vi "combineZip.vi"(0 "basicPath":path, 5 "zipArray":path[](array[path]), 7 "combinedZip":path, 9 "status":refnum<vi>, 11 "错误输入":errorcluster) -> (4 "combinedZip out":path, 15 "error IO":errorcluster)   [LabVIEW 2011]
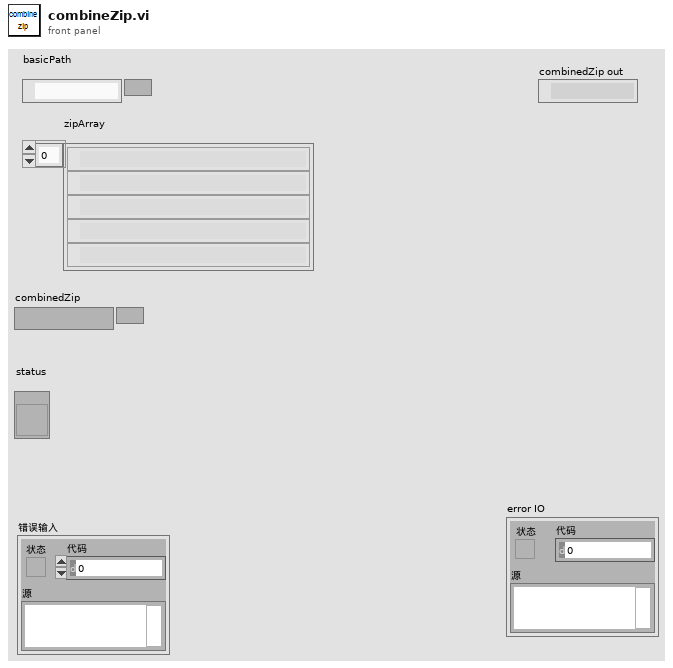
[diagram p1: front panel]
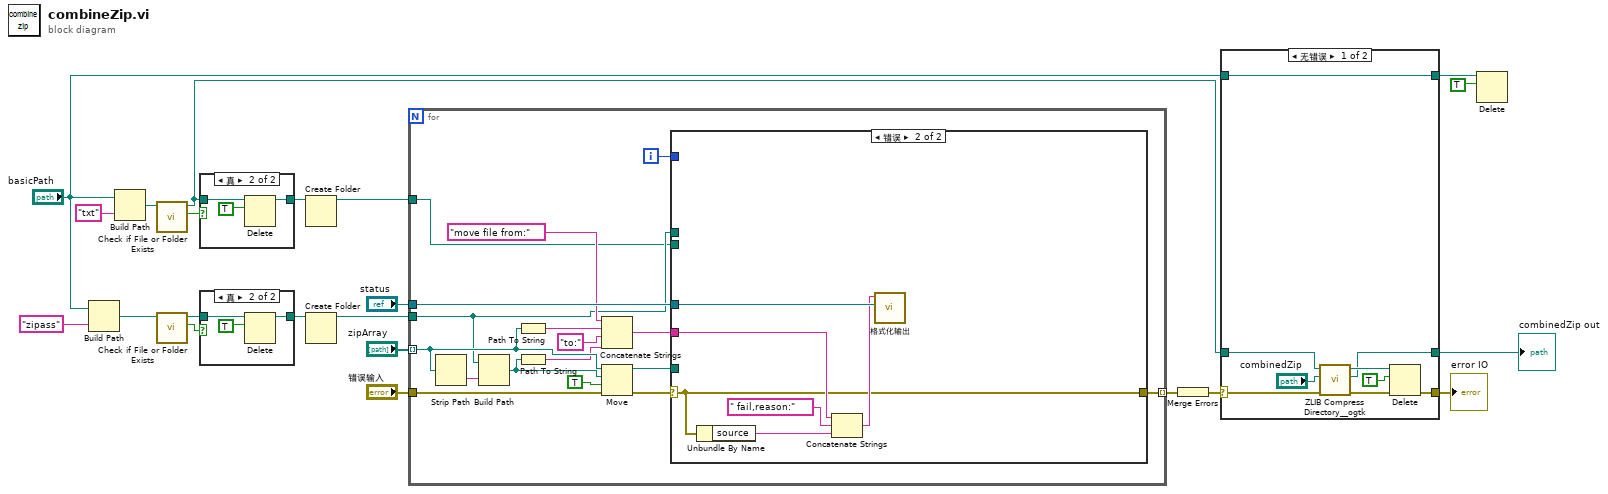
[diagram p0: block diagram]
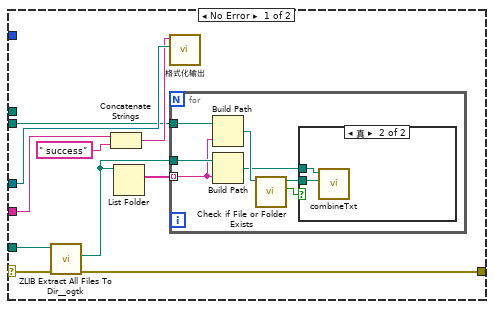
[diagram p5: hidden frame]
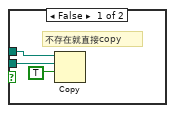
[diagram p6: hidden frame]
diagram:
  n1 = Build Path(base path="basicPath", name or relative path="zipass" ("名称或相对路径")) -> (appended path=w16:path)
  n2 = Build Path(base path="basicPath", name or relative path="txt" ("名称或相对路径")) -> (appended path=w11:path)
  n3 = call <vilib>:"Check if File or Folder Exists.vi"("path"=w11) -> ("file or folder exists?"=w13:bool, "dup path"=w7:path)  [unwired: 8 in, 1 out]
  n4 = call <vilib>:"Check if File or Folder Exists.vi"("path"=w16) -> ("file or folder exists?"=w20:bool, "dup path"=w19:path)  [unwired: 8 in, 1 out]
  n5 = case shown="真" w13 {
    tunnel: w7 -> [w23 w26]
    tunnel: [w23 w24] -> w12
    frame False {
    }
    frame True {
      n6 = Delete(path (use dialog)=w26, entire hierarchy (F)=TRUE ("整个层次结构(F)")) -> (deleted path=w24:path)  [unwired: 3 in, 2 out]
    }
  }
  n7 = case shown="真" w20 {
    tunnel: w19 -> [w27 w30]
    tunnel: [w27 w28] -> w18
    frame False {
    }
    frame True {
      n8 = Delete(path (use dialog)=w30, entire hierarchy (F)=TRUE ("整个层次结构(F)")) -> (deleted path=w28:path)  [unwired: 3 in, 2 out]
    }
  }
  n9 = Create Folder(path (use dialog)=w12) -> (created path=w10:path)  [unwired: 2 in, 2 out]
  n10 = Create Folder(path (use dialog)=w18) -> (created path=w17:path)  [unwired: 2 in, 2 out]
  n11 = for {
    tunnel: "zipArray" -> [w42] mode=indexing
    tunnel: w17 -> [w34]
    tunnel: "status" -> [w43]
    tunnel: "错误输入" -> [w35]
    tunnel: [w32] -> w9 mode=indexing
    tunnel: w10 -> [w31]
    i -> [w33]
    n12 = Strip Path(path=w42) -> (name=w47:string)  [unwired: 1 out]
    n13 = Build Path(base path=w34, name or relative path=w47) -> (appended path=w41:path)
    n14 = Path To String(path=w42) -> (string=w39:string)
    n15 = Path To String(path=w41) -> (string=w37:string)
    n16 = Concatenate Strings("move file from:" ("字符串"), w39, "to:" ("字符串"), w37) -> (w36:string)
    n17 = Move(source path=w42, error in=w35, 9:TRUE ("覆盖(F)"), 10:w41) -> (error out=w45:errorcluster, 3:w44:path)  [unwired: 1 in, 1 out]
    n18 = case shown="错误" w45 {
      selector: w45 -> [w52 w70]
      tunnel: w44 -> [w57 _]
      tunnel: w43 -> [w56 w72]
      tunnel: w36 -> [w55 w75]
      tunnel: w34 -> [_ _]
      tunnel: w33 -> [_ _]
      tunnel: [w51 w70] -> w32
      tunnel: w31 -> [w48 _]
      frame No Error {
        n19 = call <userlib>:"ZLIB Extract All Files To Dir__ogtk.vi"("error in (no error)"=w52, "archive name (file dialog)"=w57) -> ("error out"=w51:errorcluster, "root directory out"=w49:path)  [unwired: 7 in, 1 out]
        n20 = Concatenate Strings(w55, " success" ("字符串")) -> (w53:string)
        n21 = List Folder(path=w49) -> (filenames=w50:string[])  [unwired: 3 in, 3 out]
        n22 = call "格式化输出.vi"("字符串引用"=w56, "字符串"=w53) -> ()  [unwired: 9 in, 1 out]
        n23 = for {
          tunnel: w50 -> [w62] mode=indexing
          tunnel: w49 -> [w64]
          tunnel: w48 -> [w63]
          n24 = Build Path(base path=w63, name or relative path=w62) -> (appended path=w61:path)
          n25 = Build Path(base path=w64, name or relative path=w62) -> (appended path=w59:path)
          n26 = call <vilib>:"Check if File or Folder Exists.vi"("path"=w61) -> ("file or folder exists?"=w60:bool, "dup path"=w58:path)  [unwired: 8 in, 1 out]
          n27 = case shown="真" w60 {
            tunnel: w59 -> [w67 w69]
            tunnel: w58 -> [w66 w68]
            frame False {
              # "不存在就直接copy"
              n28 = Copy(9:TRUE ("覆盖(F)"), 10:w66, 11:w67) -> ()  [unwired: 2 in, 3 out]
            }
            frame True {
              n29 = call "combineTxt.vi"("parentPath"=w68, "childPath"=w69) -> ()  [unwired: 9 in, 1 out]
            }
          }
        }
      }
      frame Error {
        n30 = Unbundle By Name(w70) -> ("source"=w73:string)
        n31 = Concatenate Strings(w75, " fail,reason:" ("字符串"), w73) -> (w71:string)
        n32 = call "格式化输出.vi"("字符串引用"=w72, "字符串"=w71) -> ()  [unwired: 9 in, 1 out]
      }
    }
  }
  n33 = Merge Errors(w9) -> (w8:errorcluster)
  n34 = case shown="无错误" w8 {
    selector: w8 -> [w80 w86]
    tunnel: w7 -> [w84 _]
    tunnel: [w78 w86] -> w5
    tunnel: [w77 _] -> w6
    tunnel: "basicPath" -> [w76 w85]
    tunnel: [w76 w85] -> w2
    frame No Error {
      n35 = call <userlib>:"ZLIB Compress Directory__ogtk.vi"("error in (no error)"=w80, "archive name (root directory with .zip ending)"="combinedZip", "root directory (file dialog)"=w84) -> ("error out"=w79:errorcluster, "archive name out"=w77:path, "root directory out"=w82:path)  [unwired: 6 in]
      n36 = Delete(path (use dialog)=w82, entire hierarchy (F)=TRUE ("整个层次结构(F)"), error in=w79) -> (error out=w78:errorcluster)  [unwired: 2 in, 2 out]
    }
    frame Error {
    }
  }
  "combinedZip out" <- w6
  "error IO" <- w5
  n37 = Delete(path (use dialog)=w2, entire hierarchy (F)=TRUE ("整个层次结构(F)")) -> ()  [unwired: 3 in, 3 out]
